vi "Ultrasonic.vi"(0 "AIDeviceRef":T1={"DevStatus"={"status"=FALSE, "code"=0, "source"=""}, "Analog Module"=enum."Analog Module 1", "Analog Channel"=enum."Invalid"}, 5 "Scaling factor (Vcc/cm)":dbl=0.0098, 11 "error in (no error)":errorcluster) -> (4 "AIDeviceRef_Out":T1={"DevStatus"={"status"=FALSE, "code"=0, "source"=""}, "Analog Module"=enum."Analog Module 1", "Analog Channel"=enum."Invalid"}, 6 "Distance":dbl, 15 "error out":errorcluster)   [LabVIEW 2013]
uses:
  <vilib>/Rock Robotics/WPI/AnalogChannel/WPI_AnalogChannelDevRef.ctl
  <vilib>/Rock Robotics/SystemInterfaces/Typedef/FPGA_TypedefAnalogModule.ctl
  <vilib>/Rock Robotics/SystemInterfaces/AI/FPGA_AIChannel.ctl
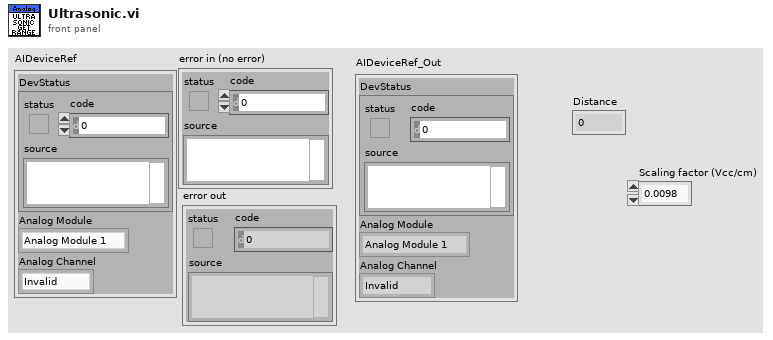
[diagram p1: front panel]
types:
  T1 = typedef "WPI_AnalogChannelDevRef.ctl" = cluster{"DevStatus":errorcluster, "Analog Module":T2, "Analog Channel":T3}
  T2 = typedef "FPGA_TypedefAnalogModule.ctl" = enum16{"Analog Module 1", "Analog Module 2"}
  T3 = typedef "FPGA_AIChannel.ctl" = enum8{"AI 1", "AI 2", "AI 3", "AI 4", "AI 5", "AI 6", "AI 7", "AI 8", "Invalid"}
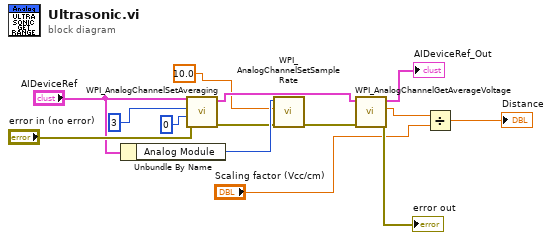
[diagram p0: block diagram]
diagram:
  n1 = Unbundle By Name("AIDeviceRef") -> ("Analog Module"=w11:T2)
  n2 = call <vilib>:"WPI_AnalogChannelSetAveraging.vi"("error in (no error)"="error in (no error)", "OversampleBits"=u8 0, "AverageBits"=3, "AIDeviceRef"="AIDeviceRef") -> ("error out"=w10:errorcluster, "AIDeviceRef"=w8:T1)  [unwired: 6 in]
  n3 = call <vilib>:"WPI_AnalogChannelSetSampleRate.vi"("error in (no error)"=w10, "Samples Per Second"=10.0, "Analog Module (Module 1)"=w11) -> ("error out"=w9:errorcluster)  [unwired: 7 in, 1 out]
  n4 = call <vilib>:"WPI_AnalogChannelGetAverageVoltage.vi"("error in (no error)"=w9, "AIDeviceRef"=w8) -> ("error out"=→"error out":errorcluster, "Voltage"=w3:dbl, "AIDeviceRef"=→"AIDeviceRef_Out":T1)  [unwired: 7 in]
  n5 = Divide(x=w3, y="Scaling factor (Vcc/cm)") -> (x/y=→"Distance":dbl)
